vi "Created Aliases.vi"(11 "Base Actor in":refnum<class "Base Actor.lvclass">) -> (2 "Created Aliases":T1)   [LabVIEW 2021, in "jettl.lvlib" / "Actor.lvlib" / "Base Actor.lvclass"]
uses:
  Base Actor.lvclass
  Created Aliases.ctl
  Base Actor.lvclass/Base Actor.ctl
  Actor.lvlib
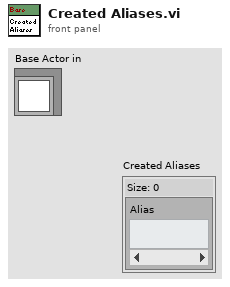
[diagram p1: front panel]
types:
  T1 = typedef "jettl.lvlib/Actor.lvlib/Created Aliases.ctl" = set{string}
  T2 = typedef "jettl.lvlib/Actor.lvlib/Alias to Created Attributes.ctl" = map{string, T3}
  T3 = typedef "jettl.lvlib/Actor.lvlib/Attributes.ctl" = cluster{"Alias":string, "Address":refnum<user-event>, "Implemented Msgs":T4, "Path":path}
  T4 = typedef "jettl.lvlib/Actor.lvlib/Implemented Msgs.ctl" = set{refnum<class "Msg.lvclass">}
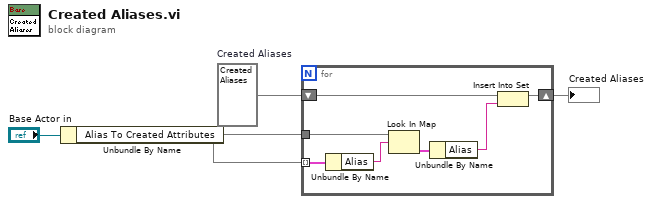
[diagram p0: block diagram]
diagram:
  w3 = T1 {}  # Created Aliases
  n1 = Unbundle By Name("Base Actor in") -> ("Alias To Created Attributes"=w1:T2)
  n2 = for {
    shift-right: [w10] -> w2
    shift-left: w3 -> [w11]
    tunnel: w1 -> [w9]
    tunnel: w1 -> [w6] mode=indexing
    n3 = Unbundle By Name(w6) -> ("Alias"=w5:string)
    n4 = Look In Map(map=w9, key=w5) -> (value=w8:T3)  [unwired: 1 in, 1 out]
    n5 = Unbundle By Name(w8) -> ("Alias"=w7:string)
    n6 = Insert Into Set(10:w7, 11:w11) -> (3:w10:T1)  [unwired: 1 out]
  }
  "Created Aliases" <- w2
